vi "Vi 2.vi"() -> ()   [LabVIEW 2010]
panel:
  in  "stop":bool
  out "Divisiòn":dbl
  out "Multiplicaciòn":dbl
  out "Resta":dbl
  out "Suma":dbl
  in  "?":dbl
  in  "Inserte sus dos nùmeros enteros":dbl
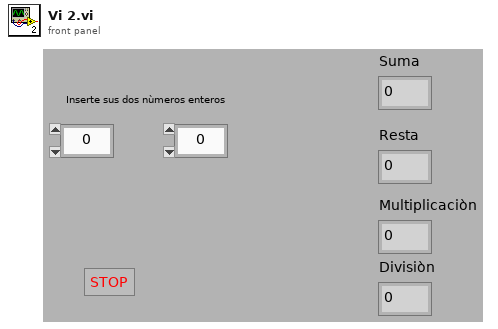
[diagram p1: front panel]
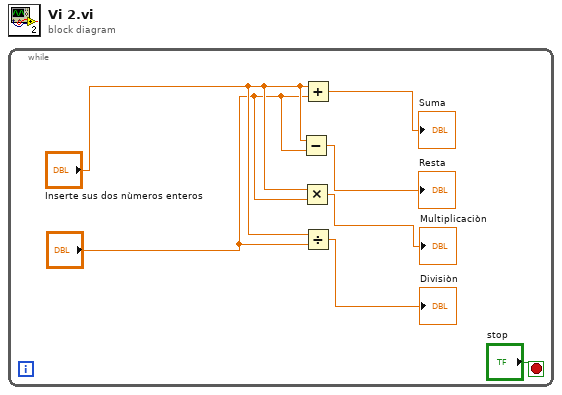
[diagram p0: block diagram]
diagram:
  n1 = while {
    stop <- "stop" stop-if-true
    n2 = Subtract(x="Inserte sus dos nùmeros enteros", y="?") -> (x-y=→"Resta":dbl)
    n3 = Multiply(x="Inserte sus dos nùmeros enteros", y="?") -> (x*y=→"Multiplicaciòn":dbl)
    n4 = Add(x="Inserte sus dos nùmeros enteros", y="?") -> (x+y=→"Suma":dbl)
    n5 = Divide(x="Inserte sus dos nùmeros enteros", y="?") -> (x/y=→"Divisiòn":dbl)
  }
